vi "File handling - Generate File Headers.vi"(8 "error in (no error)":errorcluster) -> (0 "error out":errorcluster, 1 "Analog Variables":T1[](array[typedef]), 2 "Column Units":string[](array[string]), 3 "Column Names":string[](array[string]), 5 "Digital Variables":T2[](array[typedef]))   [LabVIEW 2011]
uses:
  emi cndiates/bin File/Log emibin/Log11/Ch Info u8 std.ctl
  emi cndiates/bin File/Log emibin/Log11/Ch Info dbl.ctl
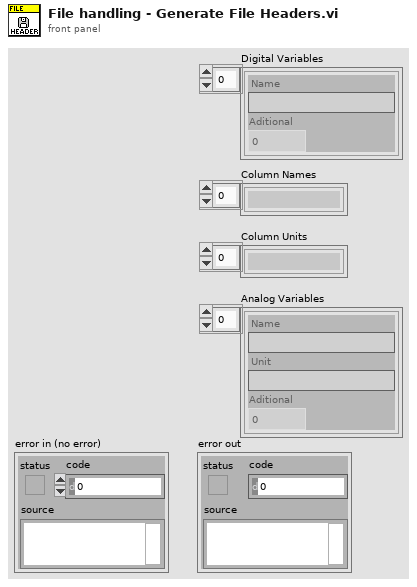
[diagram p1: front panel]
types:
  T1 = typedef "Ch Info dbl.ctl" = cluster{"Name":string, "Unit":string, "Aditional":i32}
  T2 = typedef "Ch Info u8 std.ctl" = cluster{"Name":string, "Aditional":i32}
  T3 = typedef "Fixed Analog Channel Definition.ctl" = cluster{"ID":u16, "Name":string, "Quantity":T4, "Unit":string, "Maximum upd":T5, "Comment":string, "Help file Name":string, "Help file Section ":string, "Category":T6, "User adjustable Scaling":bool, "Default Scaling":T7, "Default Unit":i32, "Classification":T8}
  T4 = typedef "Quantity enum.ctl" = enum16{"NA", "Acceleration", "Angle", "Current", "Force", "Distance", "Pressure", "Resistance", "Rotational Speed", "Speed", "Temperature", "Tension", "Torque", "Voltage", "Weight"}
  T5 = typedef "Update frequensies.ctl" = enum16{"2 Hz", "1 Hz", "0.1 Hz"}
  T6 = typedef "Channel catagory Enum.ctl" = enum16{"No Category", "Power", "Temperature", "Pressure"}
  T7 = typedef "Scaling.ctl" = cluster{"Gain":dbl, "Offset":dbl}
  T8 = typedef "Channel Classification Enum.ctl" = enum16{"Basic", "Advanced", "Expert", "Unused"}
  T9 = typedef "Fixed Digital Channel Definition.ctl" = cluster{"ID":u16, "Name":string, "NA Text":string, "Off Text":string, "On Text":string, "Maximum upd":T5, "Comment":string, "Help file Name":string, "Help file Section ":string, "Catagory":T6, "In use":bool}
  T10 = typedef "User Setting Analog Channel Bg.ctl" = cluster{"Scaling":T7, "Limits and responces":T11, "Allow Graph selection by user":bool, "Unit":u16}
  T11 = typedef "Alarm Setup Analog.ctl" = cluster{"Technical Error(NA)":T12, "LL":T12, "L":T12, "H":T12, "HH":T12, "Limits":T14}
  T12 = typedef "Alarm Responce.ctl" = cluster{"Action":T13, "Alarm":bool}
  T13 = typedef "Action List.ctl" = enum16{"No Action", "Stop Motor", "Turn Off HV"}
  T14 = typedef "Limits.ctl" = cluster{"LL":dbl, "L":dbl, "H":dbl, "HH":dbl}
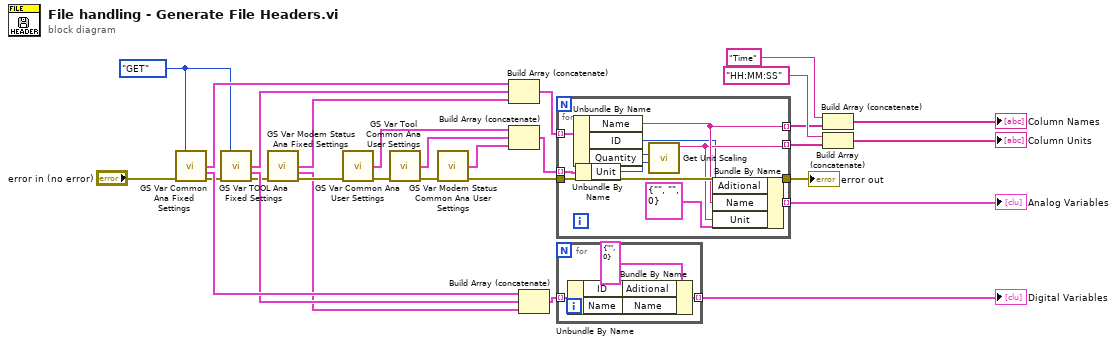
[diagram p0: block diagram]
diagram:
  w15 = enum16{"GET", "SET"}."GET" ("Action(GET)")
  n1 = call "GS Var Common Ana Fixed Settings.vi"("Action(GET)"=w15, "error in (no error)"="error in (no error)") -> ("Common Analog Var Fixed out"=w18:T3[], "Common Digital var Fixed"=w22:T9[], "error out"=w16:errorcluster)  [unwired: 11 in]
  n2 = call "GS Var TOOL Ana Fixed Settings.vi"("Action(GET)"=w15, "error in (no error)"=w16) -> ("Tool Analog var Fixed out"=w19:T3[], "Tool Digital Var Fixed out"=w21:T9[], "error out"=w4:errorcluster)  [unwired: 11 in]
  n3 = call "GS Var Modem Status Ana Fixed Settings.vi"("error in (no error)"=w4) -> ("Modem Status Analog var Fixed out"=w2:T3[], "Modem Status Digital Var Fixed out"=w1:T9[], "error out"=w3:errorcluster)  [unwired: 12 in]
  n4 = call "GS Var Common Ana User Settings.vi"("error in (no error)"=w3) -> ("Common Analog var User set out"=w24:T10[], "error out"=w23:errorcluster)  [unwired: 12 in, 1 out]
  n5 = call "GS Var Tool Common Ana User Settings.vi"("error in (no error)"=w23) -> ("Tool Analog var User settigns out"=w25:T10[], "error out"=w7:errorcluster)  [unwired: 12 in, 1 out]
  n6 = call "GS Var Modem Status Common Ana User Settings.vi"("error in (no error)"=w7) -> ("Modem Status Analog var User settigns out"=w6:T10[], "error out"=w5:errorcluster)  [unwired: 12 in, 1 out]
  n7 = Build Array (concatenate)(w18, w19, w2) -> (w20:T3[])
  n8 = Build Array (concatenate)(w24, w25, w6) -> (w26:T10[])
  n9 = Build Array (concatenate)(w22, w21, w1) -> (w17:T9[])
  n10 = for {
    tunnel: w5 -> [w38]
    tunnel: w20 -> [w39] mode=indexing
    tunnel: [w36] -> w9 mode=indexing
    tunnel: [w31] -> w10 mode=indexing
    tunnel: [w38] -> w14
    tunnel: [w35] -> w27 mode=indexing
    tunnel: w26 -> [w34] mode=indexing
    n11 = Unbundle By Name(w39) -> ("Name"=w36:string, "ID"=w30:u16, "Quantity"=w33:T4)
    n12 = Unbundle By Name(w34) -> ("Unit"=w32:u16)
    n13 = call "Get Unit Scaling.vi"("Unit Index"=w32, "Quantity"=w33) -> ("Unit"=w31:string)  [unwired: 7 in, 2 out]
    n14 = Bundle By Name(cluster=T1 {"Name"="", "Unit"="", "Aditional"=0} ("Ch Info dbl"), "Aditional"=w30, "Name"=w36, "Unit"=w31) -> (w35:T1)
  }
  "Analog Variables" <- w27
  "error out" <- w14
  n15 = for {
    tunnel: w17 -> [w44] mode=indexing
    tunnel: [w40] -> w28 mode=indexing
    n16 = Unbundle By Name(w44) -> ("ID"=w42:u16, "Name"=w41:string)
    n17 = Bundle By Name(cluster=T2 {"Name"="", "Aditional"=0} ("Ch Info u8 std"), "Aditional"=w42, "Name"=w41) -> (w40:T2)
  }
  "Digital Variables" <- w28
  n18 = Build Array (concatenate)("Time" ("Name"), w9) -> (→"Column Names":string[])
  n19 = Build Array (concatenate)("HH:MM:SS" ("Name"), w10) -> (→"Column Units":string[])
